vi "User Interface.vi"(8 "error in":errorcluster, 11 "User Interface in":refnum<class "User Interface.lvclass">) -> (0 "error out":errorcluster, 3 "User Interface out":refnum<class "User Interface.lvclass">)   [LabVIEW 2020, in "RDMA.lvlib" / "RDMA Transfer Rx User Interface.lvclass"]
uses:
  RDMA Transfer Rx User Interface.lvclass
  DSF Core.lvlibp/Classes/User Interface/User Interface.lvclass
  Configuration/Rx Transfer/RDMA Transfer Rx Configuration.lvclass
  C:/dev/niveristand-data-sharing-framework-custom-device-plugins/Components/DSF Core.lvlibp/Classes/Configuration/Configuration.lvclass
  C:/dev/niveristand-data-sharing-framework-custom-device-plugins/Components/Transceivers/RDMA/Configuration/Rx Transfer/RDMA Transfer Rx Configuration.lvclass
panel:
  in  "Decimation":u16
  in  "Local Address":string
  in  "Local Port":u16
  # "RDMA Plugin Settings"
  # "* The local address field must be in IP dot notation. \n   Example: 10.0.53.23"
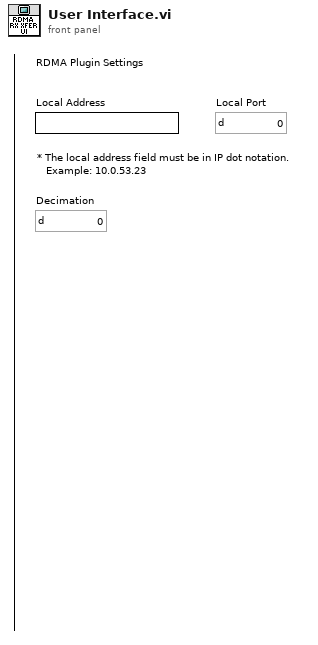
[diagram p1: front panel]
types:
  T1 = typedef "RDMA.lvlib/RDMA Transfer Rx Configuration.lvclass/Rx Transfer Settings.ctl" = cluster{"local address":u32, "local port":u16, "decimation":u16}
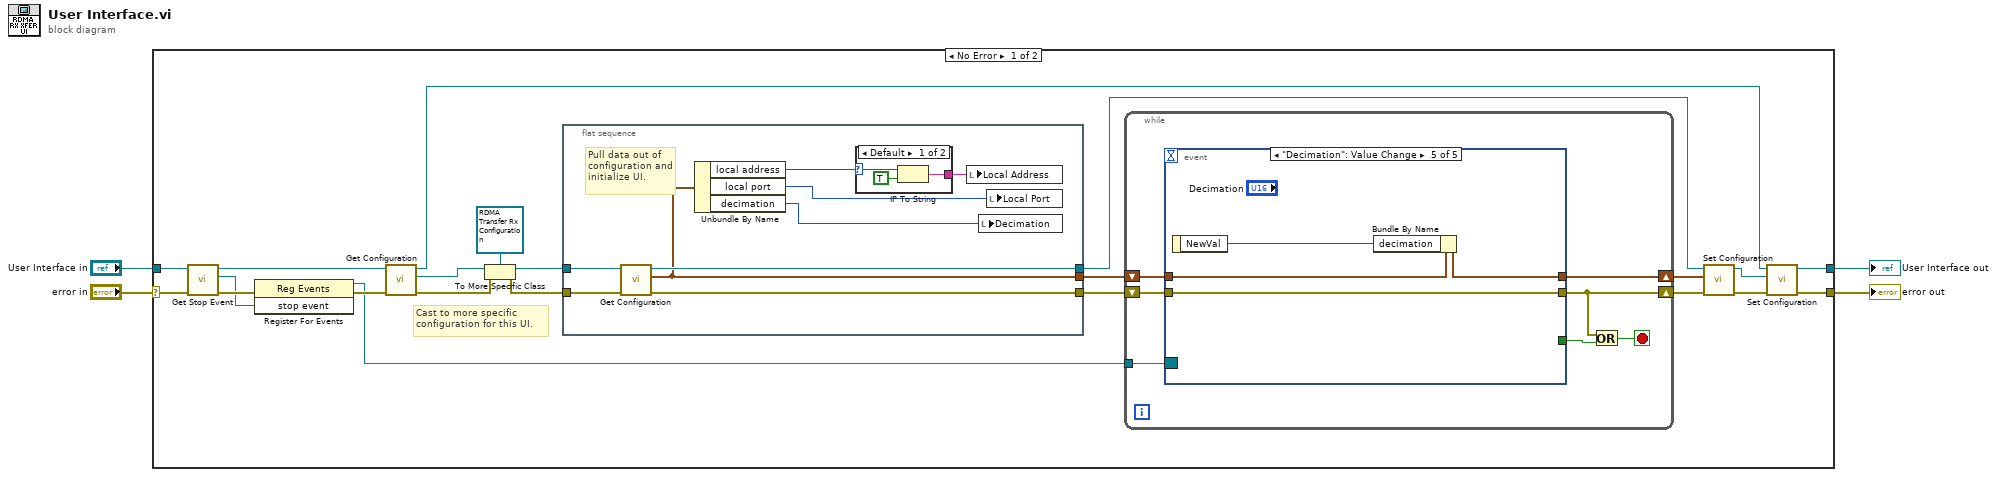
[diagram p0: block diagram]
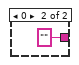
[diagram p2: hidden frame]
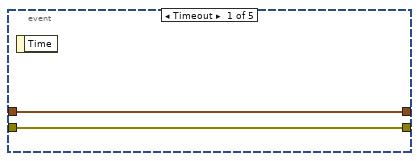
[diagram p3: hidden frame]
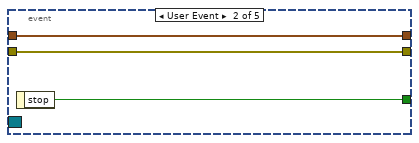
[diagram p4: hidden frame]
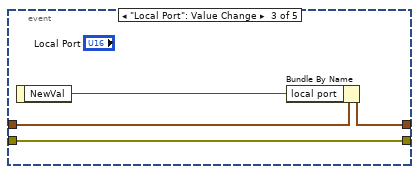
[diagram p5: hidden frame]
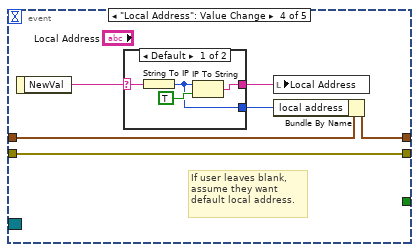
[diagram p6: hidden frame]
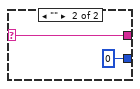
[diagram p7: hidden frame]
diagram:
  n1 = case shown="No Error" "error in" {
    selector: "error in" -> [w23 w73]
    tunnel: [w14 w73] -> w4
    tunnel: "User Interface in" -> [w22 w72]
    tunnel: [w13 w72] -> w1
    frame No Error {
      # "Cast to more specific configuration for this UI."
      n2 = call "Get Stop Event.vi"("error in (no error)"=w23, "User Interface in"=w22) -> ("error out"=w21:errorcluster, "stop event"=w20:refnum<user-event>, "User Interface out"=w19:refnum<class "User Interface.lvclass">)  [unwired: 7 in]
      n3 = register-events(error in=w21, w20) -> (reference out=w17:refnum<event-registration>, error out=w18:errorcluster)  [unwired: 1 in]
      n4 = call "Get Configuration.vi"("error in (no error)"=w18, "User Interface in"=w19) -> ("error out"=w16:errorcluster, "configuration"=w15:refnum<class "Configuration.lvclass">, "User Interface out"=w12:refnum<class "User Interface.lvclass">)  [unwired: 7 in]
      n5 = To More Specific Class(target class=refnum<class "RDMA Transfer Rx Configuration.lvclass"> refnum ("DSF Core.lvlib:UDP Transfer Rx Configuration.lvclass"), reference=w15, error in=w16) -> (specific class reference=w26:refnum<class "RDMA Transfer Rx Configuration.lvclass">, error out=w24:errorcluster)
      n6 = flat-sequence {
        tunnel: [w33] -> w25
        tunnel: w24 -> [w35]
        tunnel: w26 -> [w34]
        tunnel: [w31] -> w6
        tunnel: [w30] -> w10
        frame #0 {
          # "Pull data out of configuration and initialize UI."
          n7 = call "Get Configuration.vi"("error in"=w35, "RDMA Transfer Rx Configuration in"=w34) -> ("error out"=w33:errorcluster, "transfer settings"=w30:T1, "RDMA Transfer Rx Configuration out"=w31:refnum<class "RDMA Transfer Rx Configuration.lvclass">)  [unwired: 7 in]
          n8 = Unbundle By Name(w30) -> ("local address"=w29:u32, "local port"=w28:u16, "decimation"=w27:u16)
          n9 = case shown="Default" w29 {
            selector: w29 -> [w36 _]
            tunnel: [w38 "" ("name")] -> w32
            frame Default {
              n10 = IP To String(1:TRUE ("dot notation? (F)"), 2:w36) -> (0:w38:string)
            }
            frame 0 {
            }
          }
          n11 = local write "Local Address"(w32) -> ()
          n12 = local write "Decimation"(w27) -> ()
          n13 = local write "Local Port"(w28) -> ()
        }
      }
      n14 = while {
        tunnel: w17 -> [w46]
        shift-right: [w44] -> w9
        shift-left: w25 -> [w45]
        shift-right: [w40] -> w7
        shift-left: w10 -> [w41]
        stop <- w43 stop-if-true
        n15 = event shown="[4] \"Decimation\": Value Change" {
          selector: w46 -> [_ _ _ _ _]
          dyn-events: _ -> [_ _ _ _ _]
          timeout: _ -> [_ _ _ _ _]
          tunnel: [_ w50 _ _ _] -> w42
          tunnel: w45 -> [w48 w51 w55 w58 w68]
          tunnel: [w48 w51 w55 w58 w68] -> w44
          tunnel: w41 -> [w47 w49 w54 w59 w71]
          tunnel: [w47 w49 w53 w61 w70] -> w40
          event Timeout {
            n16 = event-data() -> ()  [unwired: 1 in, 1 out]
          }
          event User Event {
            n17 = event-data() -> ("stop"=w50:bool)  [unwired: 1 in]
          }
          event "Local Port": Value Change {
            n18 = event-data() -> ("NewVal"=w52:u16)  [unwired: 1 in]
            n19 = Bundle By Name(cluster=w54, "local port"=w52) -> (w53:T1)
          }
          event "Local Address": Value Change {
            # "If user leaves blank, assume they want default local address."
            n20 = event-data() -> ("NewVal"=w56:string)  [unwired: 1 in]
            n21 = case shown="Default" w56 {
              selector: w56 -> [w62 w66]
              tunnel: [w65 w66] -> w60
              tunnel: [w63 u32 0] -> w57
              frame Default {
                n22 = String To IP(1:w62) -> (0:w63:u32)
                n23 = IP To String(1:TRUE ("dot notation? (F)"), 2:w63) -> (0:w65:string)
              }
              frame "" {
              }
            }
            n24 = local write "Local Address"(w60) -> ()
            n25 = Bundle By Name(cluster=w59, "local address"=w57) -> (w61:T1)
          }
          event "Decimation": Value Change {
            n26 = event-data() -> ("NewVal"=w69:u16)  [unwired: 1 in]
            n27 = Bundle By Name(cluster=w71, "decimation"=w69) -> (w70:T1)
          }
        }
        n28 = Or(x=w44, y=w42) -> (x .or. y?=w43:bool)
      }
      n29 = call "Set Configuration.vi"("error in"=w9, "transfer settings"=w7, "RDMA Transfer Rx Configuration in"=w6) -> ("error out"=w8:errorcluster, "RDMA Transfer Rx Configuration out"=w5:refnum<class "RDMA Transfer Rx Configuration.lvclass">)  [unwired: 7 in]
      n30 = call "Set Configuration.vi"("error in (no error)"=w8, "configuration"=w5, "User Interface in"=w12) -> ("error out"=w14:errorcluster, "User Interface out"=w13:refnum<class "User Interface.lvclass">)  [unwired: 7 in]
    }
    frame Error {
    }
  }
  "error out" <- w4
  "User Interface out" <- w1
